vi "Get Level.vi"(8 "error in":errorcluster, 11 "LogRecord in":refnum<class "LogRecord.lvclass">) -> (0 "error out":errorcluster, 2 "Level":T1, 3 "LogRecord out":refnum<class "LogRecord.lvclass">)   [LabVIEW 2016, in "hse-logger.lvlib" / "LogRecord.lvclass"]
doc: "Returns the level of this LogRecord.\n\n____\n(c) HAMPEL SOFTWARE ENGINEERING"
uses:
  LogRecord.lvclass
  LogLevel.ctl
  LogRecord.lvclass/LogRecord.ctl
  hse-logger.lvlib
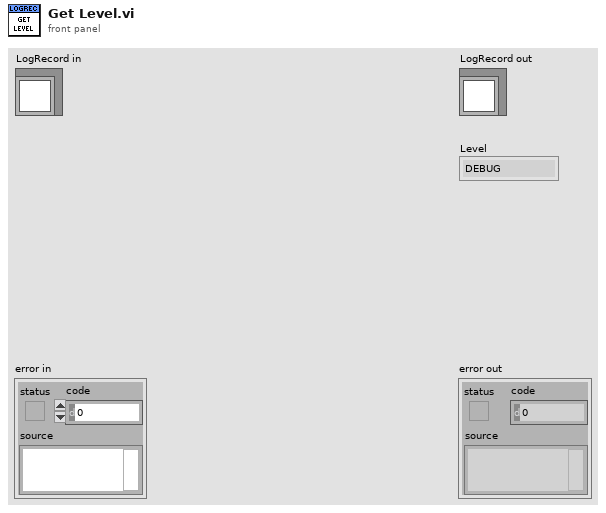
[diagram p1: front panel]
types:
  T1 = typedef "hse-logger.lvlib/LogLevel.ctl" = enum16{"DEBUG", "INFO", "WARNING", "ERROR", "CRITICAL"}
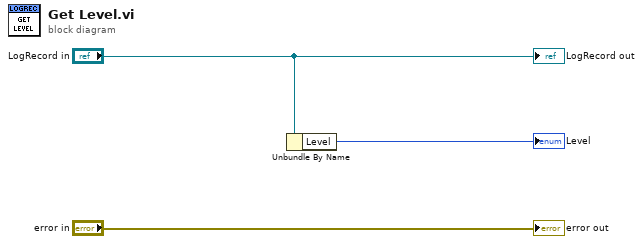
[diagram p0: block diagram]
diagram:
  n1 = Unbundle By Name("LogRecord in") -> ("Level"=→"Level":T1)
  "error out" <- "error in"
  "LogRecord out" <- "LogRecord in"
